vi "completeReceiveHealthAndStatus.vi"(8 "error in (no error)":errorcluster, 11 "Model in":refnum<class "Model.lvclass">) -> (0 "error out":errorcluster, 3 "Model out":refnum<class "Model.lvclass">)   [LabVIEW 2016, in "Model.lvclass"]
uses:
  Model.lvclass
  DataTypes/Topics/TelemetryFPGAData.ctl
  DataTypes/Topics/Parts/Timestamp.ctl
  Model.lvclass/Model.ctl
  Publisher/Publisher.lvclass/Publisher.ctl
  DataTypes/Topics/M1M3SupportTopics.lvlib
  Common_RT_HealthAndStatus/RTHealthAndStatus/RTHealthAndStatus.lvclass
  Publisher/Publisher.lvclass
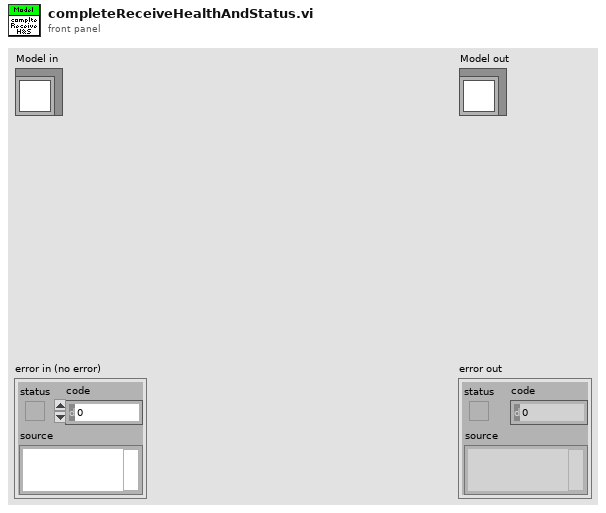
[diagram p1: front panel]
types:
  T1 = typedef "M1M3SupportTopics.lvlib/TelemetryFPGAData.ctl" = cluster{"Timestamp":T2, "ModbusSubnetATxInternalFIFOOverflow":bool, "ModbusSubnetAInvalidInstruction":bool, "ModbusSubnetAWaitForRxFrameTimeout":bool, "ModbusSubnetAStartBitError":bool, "ModbusSubnetAStopBitError":bool, "ModbusSubnetARxDataFIFOOverflow":bool, "ModbusSubnetATxByteCount":u32, "ModbusSubnetATxFrameCount":u32, "ModbusSubnetARxByteCount":u32, "ModbusSubnetARxFrameCount":u32, "ModbusSubnetBTxInternalFIFOOverflow":bool, "ModbusSubnetBInvalidInstruction":bool, "ModbusSubnetBWaitForRxFrameTimeout":bool, "ModbusSubnetBStartBitError":bool, "ModbusSubnetBStopBitError":bool, "ModbusSubnetBRxDataFIFOOverflow":bool, "ModbusSubnetBTxByteCount":u32, "ModbusSubnetBTxFrameCount":u32, "ModbusSubnetBRxByteCount":u32, "ModbusSubnetBRxFrameCount":u32, "ModbusSubnetCTxInternalFIFOOverflow":bool, "ModbusSubnetCInvalidInstruction":bool, "ModbusSubnetCWaitForRxFrameTimeout":bool, "ModbusSubnetCStartBitError":bool, "ModbusSubnetCStopBitError":bool, "ModbusSubnetCRxDataFIFOOverflow":bool, "ModbusSubnetCTxByteCount":u32, "ModbusSubnetCTxFrameCount":u32, "ModbusSubnetCRxByteCount":u32, "ModbusSubnetCRxFrameCount":u32, "ModbusSubnetDTxInternalFIFOOverflow":bool, "ModbusSubnetDInvalidInstruction":bool, "ModbusSubnetDWaitForRxFrameTimeout":bool, "ModbusSubnetDStartBitError":bool, "ModbusSubnetDStopBitError":bool, "ModbusSubnetDRxDataFIFOOverflow":bool, "ModbusSubnetDTxByteCount":u32, "ModbusSubnetDTxFrameCount":u32, "ModbusSubnetDRxByteCount":u32, "ModbusSubnetDRxFrameCount":u32, "ModbusSubnetETxInternalFIFOOverflow":bool, "ModbusSubnetEInvalidInstruction":bool, "ModbusSubnetEWaitForRxFrameTimeout":bool, "ModbusSubnetEStartBitError":bool, "ModbusSubnetEStopBitError":bool, "ModbusSubnetERxDataFIFOOverflow":bool, "ModbusSubnetETxByteCount":u32, "ModbusSubnetETxFrameCount":u32, "ModbusSubnetERxByteCount":u32, "ModbusSubnetERxFrameCount":u32, "FPGATimestamp":dbl}
  T2 = typedef "M1M3SupportTopics.lvlib/Timestamp.ctl" = dbl
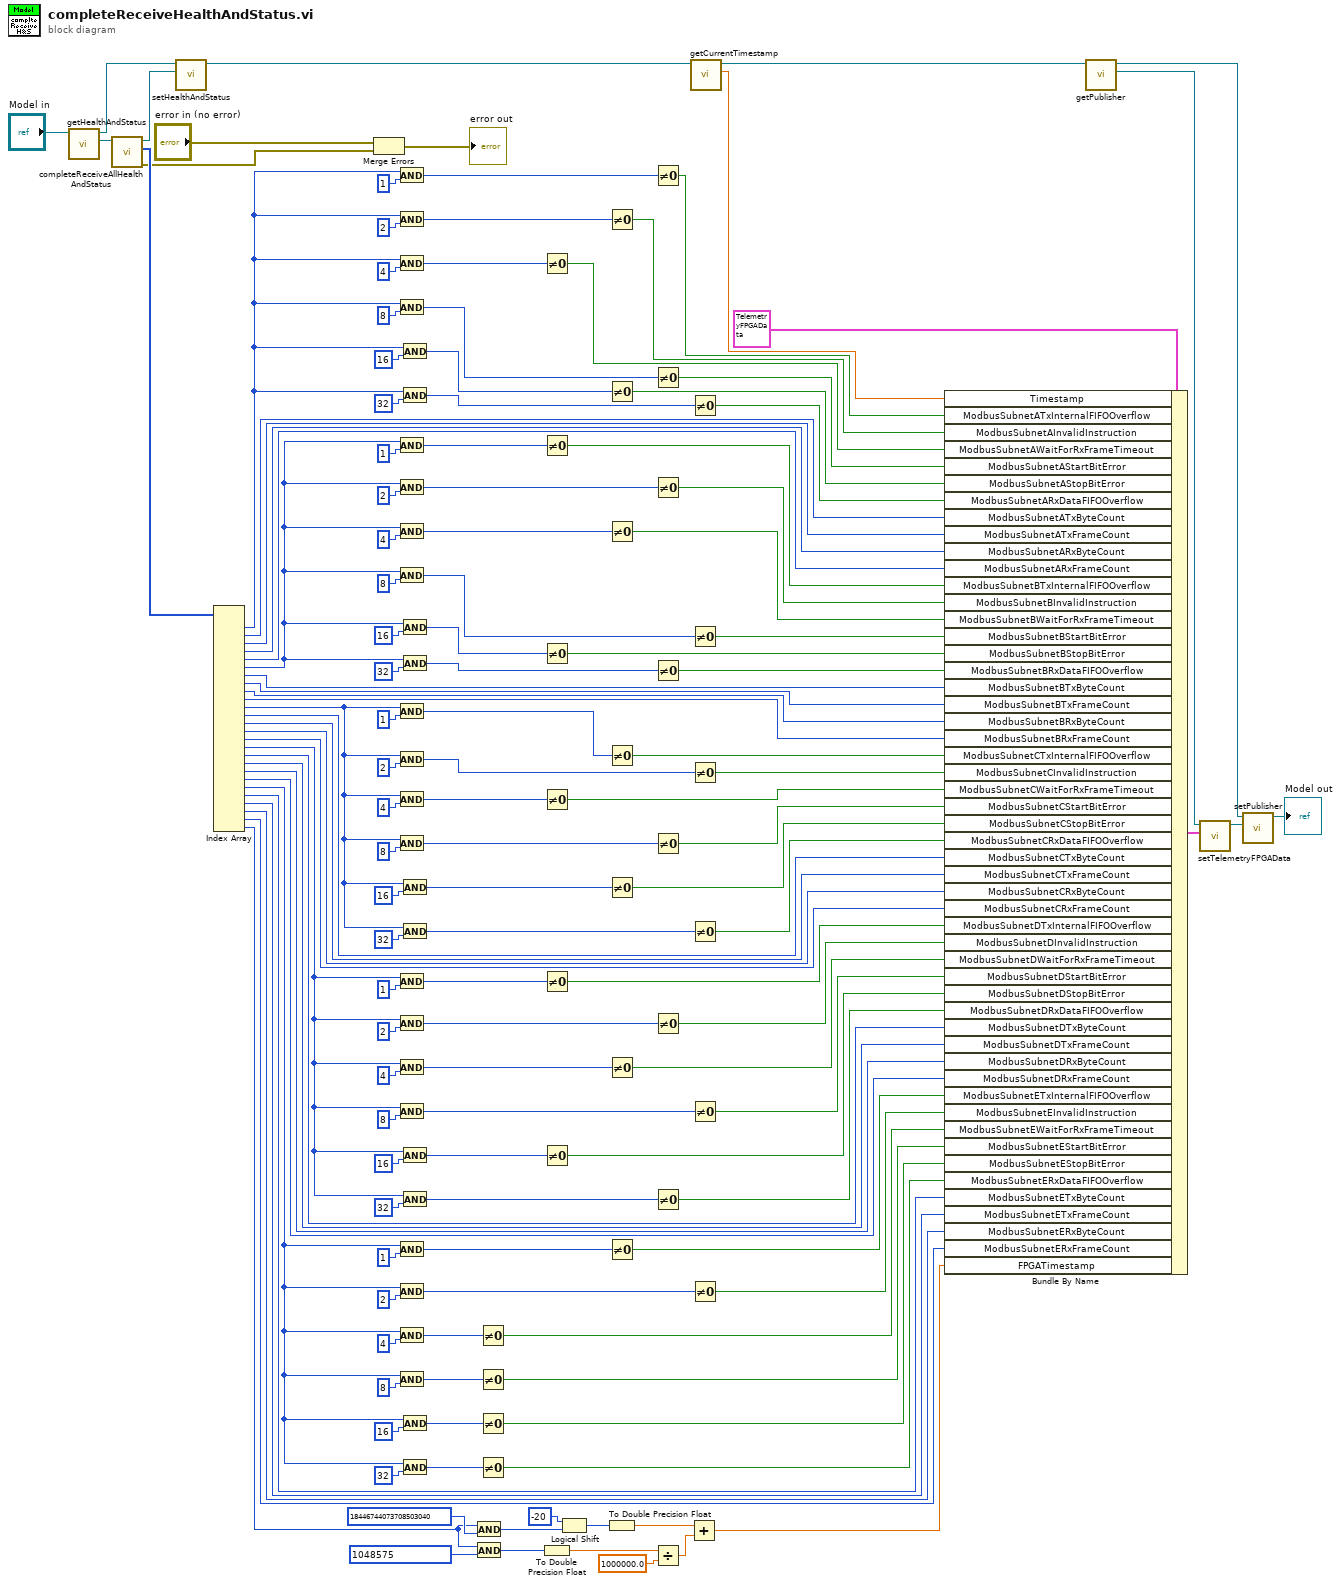
[diagram p0: block diagram]
diagram:
  n1 = call "getHealthAndStatus.vi"("Model in"="Model in") -> ("HealthAndStatus"=w14:refnum<class "RTHealthAndStatus.lvclass">, "Model out"=w11:refnum<class "Model.lvclass">)  [unwired: 9 in]
  n2 = call "completeReceiveAllHealthAndStatus.vi"("RTHealthAndStatus in"=w14) -> ("error out"=w9:errorcluster, "Data"=w13:u32[], "RTHealthAndStatus out"=w12:refnum<class "RTHealthAndStatus.lvclass">)  [unwired: 8 in]
  n3 = call "setHealthAndStatus.vi"("HealthAndStatus"=w12, "Model in"=w11) -> ("Model out"=w10:refnum<class "Model.lvclass">)  [unwired: 9 in]
  n4 = Index Array(array=w13) -> (element #1=w132:u32, element #2=w141:u32, element #3=w140:u32, element #4=w139:u32, element #5=w138:u32, element #6=w102:u32, element #7=w137:u32, element #8=w136:u32, element #9=w135:u32, element #10=w134:u32, element #11=w83:u32, element #12=w76:u32, element #13=w75:u32, element #14=w74:u32, element #15=w73:u32, element #16=w60:u32, element #17=w53:u32, element #18=w52:u32, element #19=w51:u32, element #20=w50:u32, element #21=w37:u32, element #22=w30:u32, element #23=w29:u32, element #24=w28:u32, element #25=w27:u32, element #26=w22:u32)  [unwired: 26 in]
  n5 = Merge Errors("error in (no error)", w9) -> (→"error out":errorcluster)
  n6 = And(x=w132, y=u32 1) -> (x .and. y?=w133:u32)
  n7 = And(x=w132, y=u32 2) -> (x .and. y?=w131:u32)
  n8 = And(x=w132, y=u32 4) -> (x .and. y?=w130:u32)
  n9 = And(x=w132, y=u32 8) -> (x .and. y?=w129:u32)
  n10 = And(x=w102, y=u32 1) -> (x .and. y?=w103:u32)
  n11 = And(x=w102, y=u32 2) -> (x .and. y?=w104:u32)
  n12 = And(x=w102, y=u32 4) -> (x .and. y?=w105:u32)
  n13 = And(x=w102, y=u32 8) -> (x .and. y?=w106:u32)
  n14 = And(x=w83, y=u32 1) -> (x .and. y?=w95:u32)
  n15 = And(x=w83, y=u32 2) -> (x .and. y?=w94:u32)
  n16 = And(x=w83, y=u32 4) -> (x .and. y?=w93:u32)
  n17 = And(x=w83, y=u32 8) -> (x .and. y?=w92:u32)
  n18 = And(x=w60, y=u32 1) -> (x .and. y?=w61:u32)
  n19 = And(x=w60, y=u32 2) -> (x .and. y?=w62:u32)
  n20 = And(x=w60, y=u32 4) -> (x .and. y?=w63:u32)
  n21 = And(x=w60, y=u32 8) -> (x .and. y?=w64:u32)
  n22 = And(x=w37, y=u32 1) -> (x .and. y?=w49:u32)
  n23 = And(x=w37, y=u32 2) -> (x .and. y?=w48:u32)
  n24 = And(x=w37, y=u32 4) -> (x .and. y?=w47:u32)
  n25 = And(x=w37, y=u32 8) -> (x .and. y?=w46:u32)
  n26 = And(x=w132, y=u32 16) -> (x .and. y?=w127:u32)
  n27 = And(x=w132, y=u32 32) -> (x .and. y?=w128:u32)
  n28 = And(x=w102, y=u32 16) -> (x .and. y?=w108:u32)
  n29 = And(x=w102, y=u32 32) -> (x .and. y?=w107:u32)
  n30 = And(x=w83, y=u32 16) -> (x .and. y?=w90:u32)
  n31 = And(x=w83, y=u32 32) -> (x .and. y?=w91:u32)
  n32 = And(x=w60, y=u32 16) -> (x .and. y?=w66:u32)
  n33 = And(x=w60, y=u32 32) -> (x .and. y?=w65:u32)
  n34 = And(x=w37, y=u32 16) -> (x .and. y?=w44:u32)
  n35 = And(x=w37, y=u32 32) -> (x .and. y?=w45:u32)
  n36 = And(x=w22, y=u64 18446744073708503040) -> (x .and. y?=w25:u64)
  n37 = And(x=w22, y=u64 1048575) -> (x .and. y?=w20:u64)
  n38 = Not Equal To 0?(x=w47) -> (x != 0?=w34:bool)
  n39 = Not Equal To 0?(x=w46) -> (x != 0?=w33:bool)
  n40 = Not Equal To 0?(x=w44) -> (x != 0?=w32:bool)
  n41 = Not Equal To 0?(x=w45) -> (x != 0?=w31:bool)
  n42 = Not Equal To 0?(x=w130) -> (x != 0?=w124:bool)
  n43 = Not Equal To 0?(x=w103) -> (x != 0?=w101:bool)
  n44 = Not Equal To 0?(x=w108) -> (x != 0?=w97:bool)
  n45 = Not Equal To 0?(x=w93) -> (x != 0?=w80:bool)
  n46 = Not Equal To 0?(x=w61) -> (x != 0?=w59:bool)
  n47 = Not Equal To 0?(x=w66) -> (x != 0?=w55:bool)
  n48 = To Double Precision Float(number=w20) -> (double precision float=w19:dbl)
  n49 = Logical Shift(y=i16 -20, x=w25) -> (x << y=w23:u64)
  n50 = Not Equal To 0?(x=w131) -> (x != 0?=w125:bool)
  n51 = Not Equal To 0?(x=w127) -> (x != 0?=w122:bool)
  n52 = Not Equal To 0?(x=w105) -> (x != 0?=w99:bool)
  n53 = Not Equal To 0?(x=w95) -> (x != 0?=w82:bool)
  n54 = Not Equal To 0?(x=w90) -> (x != 0?=w78:bool)
  n55 = Not Equal To 0?(x=w63) -> (x != 0?=w57:bool)
  n56 = Not Equal To 0?(x=w49) -> (x != 0?=w36:bool)
  n57 = To Double Precision Float(number=w23) -> (double precision float=w17:dbl)
  n58 = Not Equal To 0?(x=w133) -> (x != 0?=w126:bool)
  n59 = Not Equal To 0?(x=w129) -> (x != 0?=w123:bool)
  n60 = Not Equal To 0?(x=w104) -> (x != 0?=w100:bool)
  n61 = Not Equal To 0?(x=w107) -> (x != 0?=w96:bool)
  n62 = Not Equal To 0?(x=w92) -> (x != 0?=w79:bool)
  n63 = Not Equal To 0?(x=w62) -> (x != 0?=w58:bool)
  n64 = Not Equal To 0?(x=w65) -> (x != 0?=w54:bool)
  n65 = Divide(x=w19, y=1000000.0) -> (x/y=w16:dbl)
  n66 = Add(x=w17, y=w16) -> (x+y=w15:dbl)
  n67 = Not Equal To 0?(x=w128) -> (x != 0?=w121:bool)
  n68 = Not Equal To 0?(x=w106) -> (x != 0?=w98:bool)
  n69 = Not Equal To 0?(x=w94) -> (x != 0?=w81:bool)
  n70 = Not Equal To 0?(x=w91) -> (x != 0?=w77:bool)
  n71 = Not Equal To 0?(x=w64) -> (x != 0?=w56:bool)
  n72 = Not Equal To 0?(x=w48) -> (x != 0?=w35:bool)
  n73 = call "getCurrentTimestamp.vi"("Model in"=w10) -> ("Timestamp"=w142:T2, "Model out"=w6:refnum<class "Model.lvclass">)  [unwired: 8 in, 1 out]
  n74 = Bundle By Name(cluster=T1 {"Timestamp"=0.0, "ModbusSubnetATxInternalFIFOOverflow"=FALSE, "ModbusSubnetAInvalidInstruction"=FALSE, "ModbusSubnetAWaitForRxFrameTimeout"=FALSE, "ModbusSubnetAStartBitError"=FALSE, "ModbusSubnetAStopBitError"=FALSE, "ModbusSubnetARxDataFIFOOverflow"=FALSE, "ModbusSubnetATxByteCount"=0, "ModbusSubnetATxFrameCount"=0, "ModbusSubnetARxByteCount"=0, "ModbusSubnetARxFrameCount"=0, "ModbusSubnetBTxInternalFIFOOverflow"=FALSE, "ModbusSubnetBInvalidInstruction"=FALSE, "ModbusSubnetBWaitForRxFrameTimeout"=FALSE, "ModbusSubnetBStartBitError"=FALSE, "ModbusSubnetBStopBitError"=FALSE, "ModbusSubnetBRxDataFIFOOverflow"=FALSE, "ModbusSubnetBTxByteCount"=0, "ModbusSubnetBTxFrameCount"=0, "ModbusSubnetBRxByteCount"=0, "ModbusSubnetBRxFrameCount"=0, "ModbusSubnetCTxInternalFIFOOverflow"=FALSE, "ModbusSubnetCInvalidInstruction"=FALSE, "ModbusSubnetCWaitForRxFrameTimeout"=FALSE, "ModbusSubnetCStartBitError"=FALSE, "ModbusSubnetCStopBitError"=FALSE, "ModbusSubnetCRxDataFIFOOverflow"=FALSE, "ModbusSubnetCTxByteCount"=0, "ModbusSubnetCTxFrameCount"=0, "ModbusSubnetCRxByteCount"=0, "ModbusSubnetCRxFrameCount"=0, "ModbusSubnetDTxInternalFIFOOverflow"=FALSE, "ModbusSubnetDInvalidInstruction"=FALSE, "ModbusSubnetDWaitForRxFrameTimeout"=FALSE, "ModbusSubnetDStartBitError"=FALSE, "ModbusSubnetDStopBitError"=FALSE, "ModbusSubnetDRxDataFIFOOverflow"=FALSE, "ModbusSubnetDTxByteCount"=0, "ModbusSubnetDTxFrameCount"=0, "ModbusSubnetDRxByteCount"=0, "ModbusSubnetDRxFrameCount"=0, "ModbusSubnetETxInternalFIFOOverflow"=FALSE, "ModbusSubnetEInvalidInstruction"=FALSE, "ModbusSubnetEWaitForRxFrameTimeout"=FALSE, "ModbusSubnetEStartBitError"=FALSE, "ModbusSubnetEStopBitError"=FALSE, "ModbusSubnetERxDataFIFOOverflow"=FALSE, "ModbusSubnetETxByteCount"=0, "ModbusSubnetETxFrameCount"=0, "ModbusSubnetERxByteCount"=0, "ModbusSubnetERxFrameCount"=0, "FPGATimestamp"=0.0} ("TelemetryFPGAData"), "Timestamp"=w142, "ModbusSubnetATxInternalFIFOOverflow"=w126, "ModbusSubnetAInvalidInstruction"=w125, "ModbusSubnetAWaitForRxFrameTimeout"=w124, "ModbusSubnetAStartBitError"=w123, "ModbusSubnetAStopBitError"=w122, "ModbusSubnetARxDataFIFOOverflow"=w121, "ModbusSubnetATxByteCount"=w141, "ModbusSubnetATxFrameCount"=w140, "ModbusSubnetARxByteCount"=w139, "ModbusSubnetARxFrameCount"=w138, "ModbusSubnetBTxInternalFIFOOverflow"=w101, "ModbusSubnetBInvalidInstruction"=w100, "ModbusSubnetBWaitForRxFrameTimeout"=w99, "ModbusSubnetBStartBitError"=w98, "ModbusSubnetBStopBitError"=w97, "ModbusSubnetBRxDataFIFOOverflow"=w96, "ModbusSubnetBTxByteCount"=w137, "ModbusSubnetBTxFrameCount"=w136, "ModbusSubnetBRxByteCount"=w135, "ModbusSubnetBRxFrameCount"=w134, "ModbusSubnetCTxInternalFIFOOverflow"=w82, "ModbusSubnetCInvalidInstruction"=w81, "ModbusSubnetCWaitForRxFrameTimeout"=w80, "ModbusSubnetCStartBitError"=w79, "ModbusSubnetCStopBitError"=w78, "ModbusSubnetCRxDataFIFOOverflow"=w77, "ModbusSubnetCTxByteCount"=w76, "ModbusSubnetCTxFrameCount"=w75, "ModbusSubnetCRxByteCount"=w74, "ModbusSubnetCRxFrameCount"=w73, "ModbusSubnetDTxInternalFIFOOverflow"=w59, "ModbusSubnetDInvalidInstruction"=w58, "ModbusSubnetDWaitForRxFrameTimeout"=w57, "ModbusSubnetDStartBitError"=w56, "ModbusSubnetDStopBitError"=w55, "ModbusSubnetDRxDataFIFOOverflow"=w54, "ModbusSubnetDTxByteCount"=w53, "ModbusSubnetDTxFrameCount"=w52, "ModbusSubnetDRxByteCount"=w51, "ModbusSubnetDRxFrameCount"=w50, "ModbusSubnetETxInternalFIFOOverflow"=w36, "ModbusSubnetEInvalidInstruction"=w35, "ModbusSubnetEWaitForRxFrameTimeout"=w34, "ModbusSubnetEStartBitError"=w33, "ModbusSubnetEStopBitError"=w32, "ModbusSubnetERxDataFIFOOverflow"=w31, "ModbusSubnetETxByteCount"=w30, "ModbusSubnetETxFrameCount"=w29, "ModbusSubnetERxByteCount"=w28, "ModbusSubnetERxFrameCount"=w27, "FPGATimestamp"=w15) -> (w4:T1)
  n75 = call "getPublisher.vi"("Model in"=w6) -> ("Publisher"=w5:refnum<class "Publisher.lvclass">, "Model out"=w2:refnum<class "Model.lvclass">)  [unwired: 9 in]
  n76 = call "setTelemetryFPGAData.vi"("TelemetryFPGAData"=w4, "Publisher in"=w5) -> ("Publisher out"=w3:refnum<class "Publisher.lvclass">)  [unwired: 9 in]
  n77 = call "setPublisher.vi"("Publisher"=w3, "Model in"=w2) -> ("Model out"=→"Model out":refnum<class "Model.lvclass">)  [unwired: 9 in]
